vi "stop2.vi"(8 "error in (no error)":errorcluster, 9 "CameraSettings":refnum<class "CamaraSettings.lvclass">, 10 "stop":bool, 11 "Pixelfly in":refnum<class "PixelflySA.lvclass">) -> (0 "error out":errorcluster, 1 "imageSaved":bool, 2 "stopped?":bool, 3 "Pixelfly out":refnum<class "PixelflySA.lvclass">)   [LabVIEW 2011, in "PixelflySA.lvclass"]
uses:
  PixelflySA.lvclass
  Tools/CameraSettings/CamaraSettings.lvclass
  PixelflySA.lvclass/PixelflySA.ctl
  Channels.lvlib
panel:
  out "Buffer status":T1
  out "Image data":u16[][](graph)
  # "Status flags"
  # "Buffer errors"
  # "Memory usage"
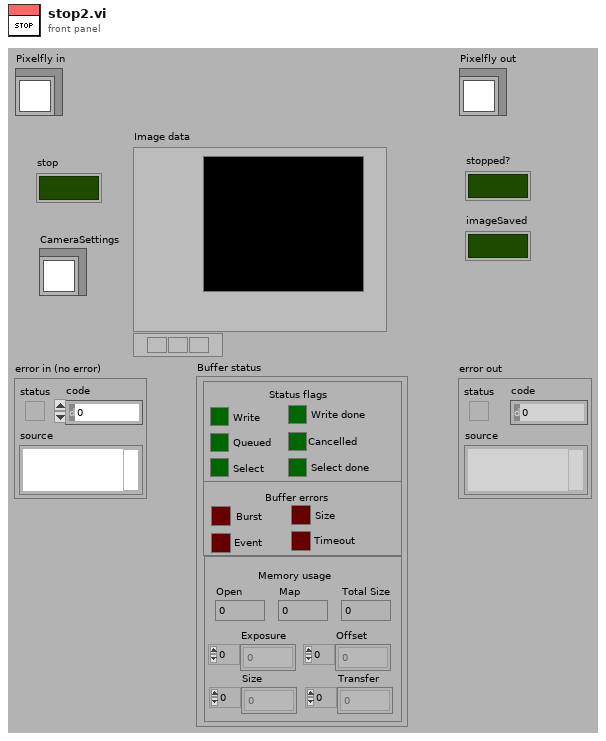
[diagram p1: front panel]
types:
  T1 = cluster{"Write":bool, "Write done":bool, "Queued":bool, "Cancelled":bool, "Select":bool, "Select done":bool, "Burst":bool, "Size":bool, "Event":bool, "Timeout":bool, "Open":i32, "Map":i32, "Exposure":i32[], "Offset":i32[], "Size":i32[], "Transfer":i32[], "Total Size":i32}
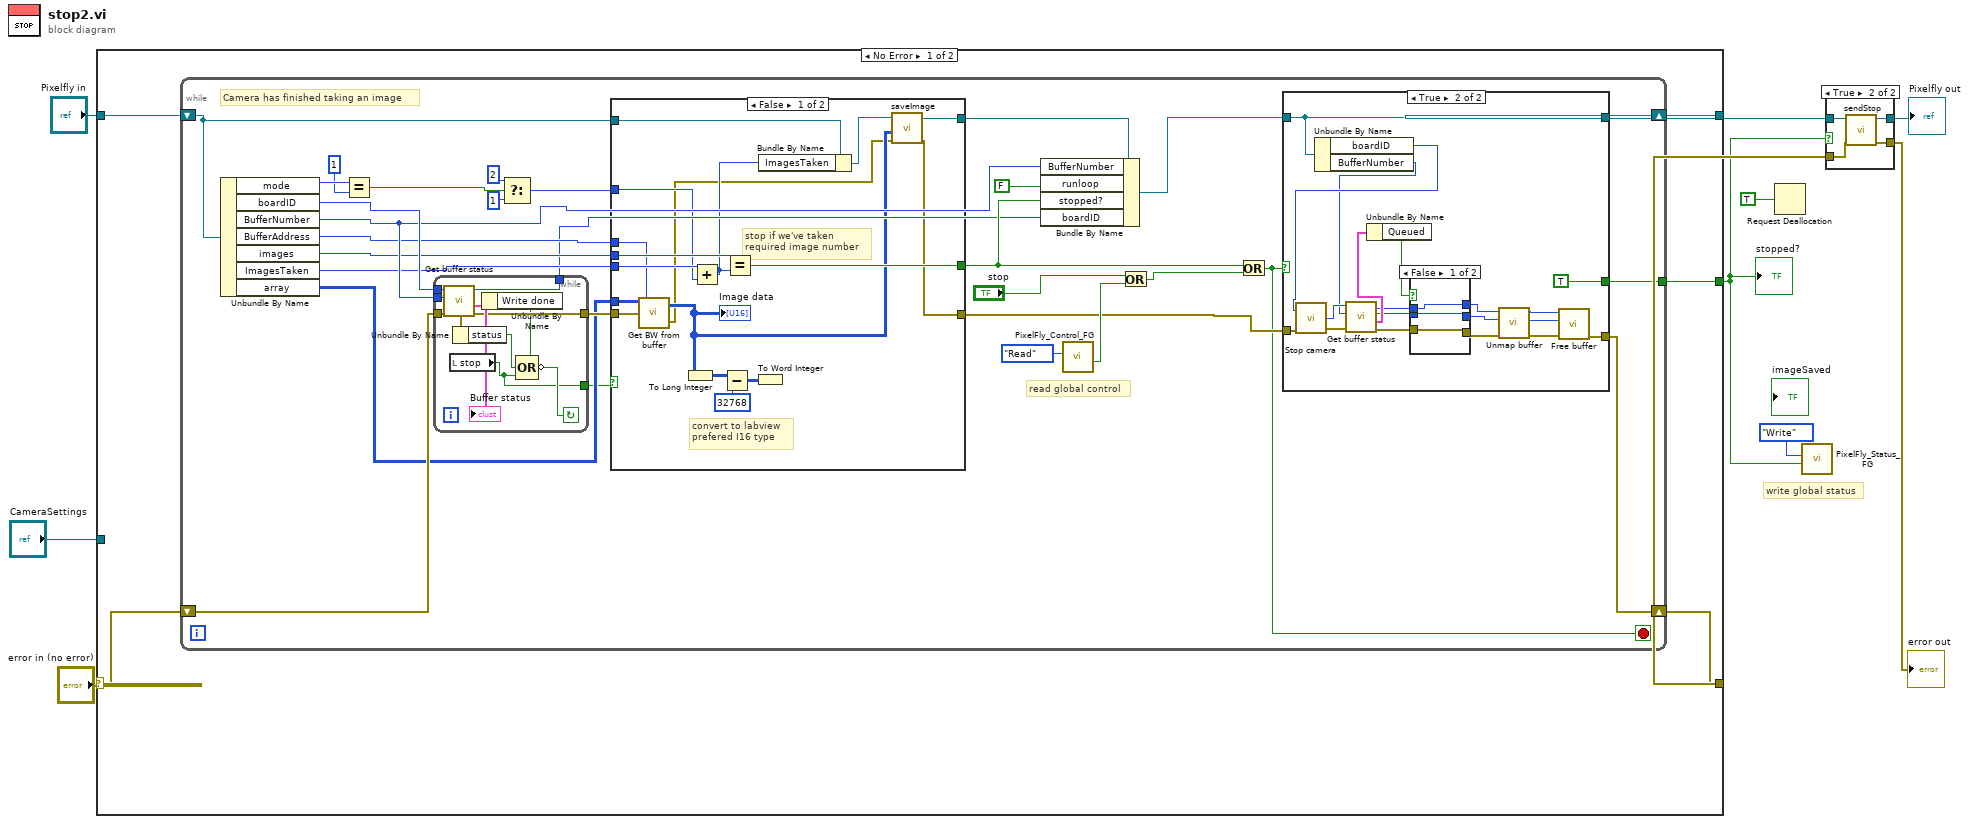
[diagram p0: block diagram]
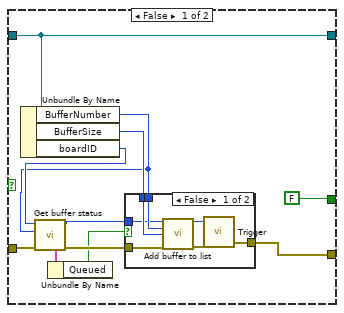
[diagram p4: hidden frame]
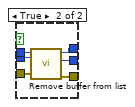
[diagram p6: hidden frame]
diagram:
  # "write global status"
  n1 = case shown="No Error" "error in (no error)" {
    selector: "error in (no error)" -> [w15 w123]
    tunnel: [w14 w123] -> w3
    tunnel: [w11 w124] -> w5
    tunnel: "Pixelfly in" -> [w12 w124]
    tunnel: "CameraSettings" -> [_ _]
    tunnel: [w13 _] -> w1
    frame No Error {
      n2 = while {
        tunnel: [w29] -> w13
        shift-right: [w18] -> w11
        shift-left: w12 -> [w19]
        shift-right: [w30] -> w14
        shift-left: w15 -> [w35]
        stop <- w21 stop-if-true
        # "Camera has finished taking an image"
        # "read global control"
        n3 = Unbundle By Name(w19) -> ("mode"=w38:u16, "boardID"=w45:i32, "BufferNumber"=w44:i32, "BufferAddress"=w41:i32, "images"=w43:i32, "ImagesTaken"=w42:i32, "array"=w17:u16[][])
        n4 = Equal?(x=w38, y=1) -> (x = y?=w36:bool)
        n5 = while {
          tunnel: w45 -> [w75]
          tunnel: w44 -> [w74]
          tunnel: w35 -> [w73]
          tunnel: [w72] -> w28
          tunnel: [w70] -> w27
          tunnel: [w66] -> w16
          stop <- w67 continue-if-true
          n6 = call <instrlib>:"Get buffer status.vi"("error in (no error)"=w73, "Buffer request"=w74, "Handle in"=w75) -> ("error out"=w70:errorcluster, "Buffer status"=w71:T1, "Handle out"=w72:i32)  [unwired: 1 in, 1 out]
          "Buffer status" <- w71
          n7 = local read "stop"() -> (w66:bool)
          n8 = Unbundle By Name(w70) -> ("status"=w68:bool)
          n9 = Unbundle By Name(w71) -> ("Write done"=w69:bool)
          n10 = Compound Arithmetic op=OR(w69, w68, w66) -> (invert w67:bool)
        }
        n11 = Select(t=2, s=w36, f=1) -> (s? t:f=w22:i32)
        n12 = case shown="False" w16 {
          selector: w16 -> [_ w63]
          tunnel: w43 -> [w62 _]
          tunnel: w42 -> [w61 _]
          tunnel: w41 -> [w60 _]
          tunnel: [w59 w63] -> w34
          tunnel: [w58 w64] -> w31
          tunnel: w27 -> [w57 w64]
          tunnel: [w52 w65] -> w25
          tunnel: w22 -> [w51 _]
          tunnel: w19 -> [w47 w65]
          tunnel: w17 -> [w46 _]
          frame False {
            # "stop if we've taken \nrequired image number"
            # "convert to labview \nprefered I16 type"
            n13 = call <instrlib>:"Get BW from buffer.vi"("error in (no error)"=w57, "Array input"=w46, "Buffer address"=w60) -> ("error out"=w48:errorcluster, "Image data"=w53:u16[][])
            "Image data" <- w53
            n14 = To Long Integer(number=w53) -> (32bit integer=w55:i32[][])
            n15 = Add(x=w61, y=w51) -> (x+y=w49:i32)
            n16 = Subtract(x=w55, y=32768) -> (x-y=w56:i32[][])
            n17 = Equal?(x=w62, y=w49) -> (x = y?=w59:bool)
            n18 = To Word Integer(number=w56) -> ()  [unwired: 1 out]
            n19 = Bundle By Name(cluster=w47, "ImagesTaken"=w49) -> (w50:refnum<class "PixelflySA.lvclass">)
            n20 = call "saveImage.vi"("error in (no error)"=w48, "I16bit image data"=w53, "Pixelfly in"=w50) -> ("error out"=w58:errorcluster, "Pixelfly out"=w52:refnum<class "PixelflySA.lvclass">)  [unwired: 7 in]
          }
          frame True {
          }
        }
        n21 = Bundle By Name(cluster=w25, "BufferNumber"=w44, "runloop"=FALSE, "stopped?"=w34, "boardID"=w28) -> (w32:refnum<class "PixelflySA.lvclass">)
        n22 = call "PixelFly_Control_FG.vi"("Action"=enum16{"Write", "Read"}."Read") -> ("stopped"=w40:bool)  [unwired: 10 in]
        n23 = Or(x="stop", y=w40) -> (x .or. y?=w33:bool)
        n24 = Or(x=w34, y=w33) -> (x .or. y?=w21:bool)
        n25 = case shown="True" w21 {
          tunnel: w32 -> [w84 w113]
          tunnel: [w84 w113] -> w18
          tunnel: w31 -> [w82 w104]
          tunnel: [w85 w110] -> w30
          tunnel: [FALSE TRUE] -> w29
          frame False {
            n26 = Unbundle By Name(w84) -> ("BufferNumber"=w80:i32, "BufferSize"=w83:i32, "boardID"=w81:i32)
            n27 = call <instrlib>:"Get buffer status.vi"("error in (no error)"=w82, "Buffer request"=w80, "Handle in"=w81) -> ("error out"=w78:errorcluster, "Buffer status"=w79:T1, "Handle out"=w77:i32)  [unwired: 1 in, 1 out]
            n28 = Unbundle By Name(w79) -> ("Queued"=w76:bool)
            n29 = case shown="False" w76 {
              tunnel: [w92 w94] -> w85
              tunnel: w83 -> [w91 _]
              tunnel: w80 -> [w90 _]
              tunnel: w78 -> [w89 w94]
              tunnel: w77 -> [w88 _]
              frame False {
                n30 = call <instrlib>:"Add buffer to list.vi"("Handle in"=w88, "Buffer in"=w90, "size"=w91, "error in (no error)"=w89) -> ("Handle out"=w87:i32, "error out"=w93:errorcluster)  [unwired: 9 in, 1 out]
                n31 = call <instrlib>:"Trigger.vi"("Handle in"=w87, "error in (no error)"=w93) -> ("error out"=w92:errorcluster)  [unwired: 2 out]
              }
              frame True {
              }
            }
          }
          frame True {
            n32 = Unbundle By Name(w113) -> ("boardID"=w103:i32, "BufferNumber"=w96:i32)
            n33 = call <instrlib>:"Stop camera.vi"("Handle in"=w103, "error in (no error)"=w104) -> ("Handle out"=w102:i32, "error out"=w105:errorcluster)  [unwired: 1 out]
            n34 = call <instrlib>:"Get buffer status.vi"("error in (no error)"=w105, "Buffer request"=w96, "Handle in"=w102) -> ("error out"=w101:errorcluster, "Buffer status"=w107:T1, "Buffer number"=w100:i32, "Handle out"=w99:i32)  [unwired: 1 in]
            n35 = Unbundle By Name(w107) -> ("Queued"=w106:bool)
            n36 = case shown="False" w106 {
              tunnel: [w116 w122] -> w98
              tunnel: [w115 w121] -> w97
              tunnel: w101 -> [w115 w120]
              tunnel: w100 -> [w114 w119]
              tunnel: w99 -> [w116 w118]
              tunnel: [w114 w117] -> w95
              frame False {
              }
              frame True {
                n37 = call <instrlib>:"Remove buffer from list.vi"("error in (no error)"=w120, "Buffer in"=w119, "Handle in"=w118) -> ("error out"=w121:errorcluster, "Buffer number"=w117:i32, "Handle out"=w122:i32)  [unwired: 2 in]
              }
            }
            n38 = call <instrlib>:"Unmap buffer.vi"("error in (no error)"=w97, "Buffer in"=w95, "Handle in"=w98) -> ("error out"=w112:errorcluster, "Buffer number"=w108:i32, "Handle out"=w111:i32)  [unwired: 2 in]
            n39 = call <instrlib>:"Free buffer.vi"("error in (no error)"=w112, "Buffer in"=w108, "Handle in"=w111) -> ("error out"=w110:errorcluster)  [unwired: 2 in, 2 out]
          }
        }
      }
    }
    frame Error {
    }
  }
  "stopped?" <- w1
  n40 = Request Deallocation(TRUE ("flag")) -> ()
  n41 = call "PixelFly_Status_FG.vi"("stop"=w1, "Action"=enum16{"Write", "Read"}."Write") -> ()  [unwired: 9 in, 1 out]
  n42 = case shown="True" w1 {
    tunnel: w5 -> [w126 w130]
    tunnel: [w126 w129] -> w4
    tunnel: w3 -> [w125 w128]
    tunnel: [w125 w127] -> w2
    frame False {
    }
    frame True {
      n43 = call "sendStop.vi"("error in (no error)"=w128, "PixelflySA in"=w130) -> ("error out"=w127:errorcluster, "PixelflySA out"=w129:refnum<class "PixelflySA.lvclass">)  [unwired: 8 in]
    }
  }
  "error out" <- w2
  "Pixelfly out" <- w4
